vi "FaultAckMultiple.vi"(6 "return immediately":bool, 8 "error in (no error)":errorcluster, 10 "axis names":string[](array[string]), 11 "controller in":refnum<k24>) -> (0 "error out":errorcluster, 3 "controller out":refnum<k24>)   [LabVIEW 2013]
uses:
  C:/GEECS/Developers Version/source/Device Driver/AerotechStage/Sample Vis/Bin/Aerotech.Ensemble.dll
  Bin/Aerotech.Ensemble.dll
  C:/GEECS/Developers Version/source/Device Driver/AerotechStage/Sample Vis/Bin/Aerotech.Ensemble.LabVIEW.dll
  Bin/Aerotech.Ensemble.LabVIEW.dll
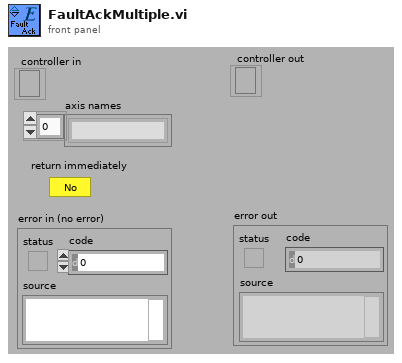
[diagram p1: front panel]
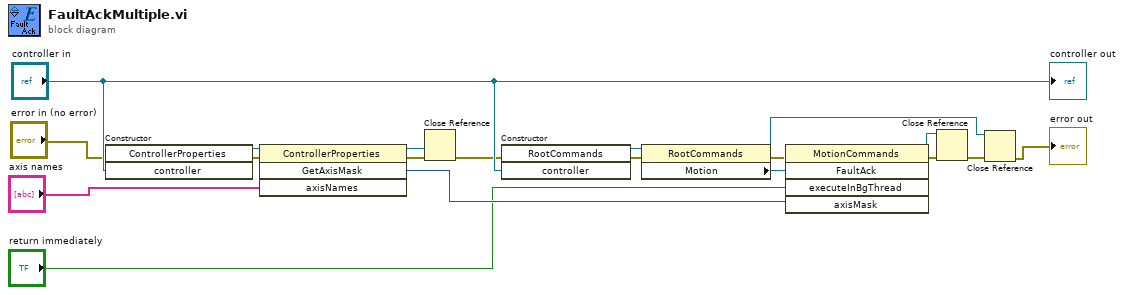
[diagram p0: block diagram]
diagram:
  n1 = constructor class="ControllerProperties"(error in="error in (no error)", "controller"="controller in") -> (reference out=w17:refnum<k24>, error out=w16:errorcluster)  [unwired: 2 in, 2 out]
  n2 = invoke class="ControllerProperties" method="GetAxisMask"(reference=w17, error in=w16, "axisNames"="axis names") -> (reference out=w14:refnum<k24>, error out=w15:errorcluster, "GetAxisMask"=w12:i32)  [unwired: 1 in, 1 out]
  n3 = Close Reference(reference=w14, error in (no error)=w15) -> (error out=w13:errorcluster)
  n4 = constructor class="RootCommands"(error in=w13, "controller"="controller in") -> (reference out=w6:refnum<k24>, error out=w5:errorcluster)  [unwired: 2 in, 2 out]
  n5 = property class="RootCommands"(reference=w6, error in=w5) -> (reference out=w1:refnum<k24>, error out=w7:errorcluster, "Motion"=w8:refnum<k24>)
  n6 = invoke class="MotionCommands" method="FaultAck"(reference=w8, error in=w7, "executeInBgThread"="return immediately", "axisMask"=w12) -> (reference out=w3:refnum<k24>, error out=w4:errorcluster)  [unwired: 1 in, 3 out]
  n7 = Close Reference(reference=w3, error in (no error)=w4) -> (error out=w2:errorcluster)
  n8 = Close Reference(reference=w1, error in (no error)=w2) -> (error out=→"error out":errorcluster)
  "controller out" <- "controller in"
